vi "Highlighted Table  rows.vi"(8 "error in":errorcluster, 10 "Number of highlighted rows":i32, 11 "Tolerance Limits Listbox":refnum<vi>) -> (0 "error out":errorcluster)   [LabVIEW 2015, in "ZenGage v3.0 UI.lvclass"]
uses:
  ZenGage v3.0 UI.lvclass
  <vilib>/Utility/miscctls.llb/LVRowAndColumnTypeDef.ctl
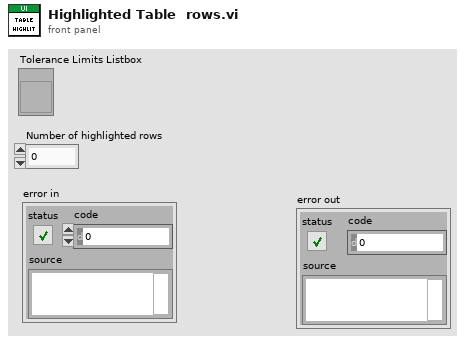
[diagram p1: front panel]
types:
  T1 = typedef "LVRowAndColumnTypeDef.ctl" = cluster{"Row":i32, "Column":i32}
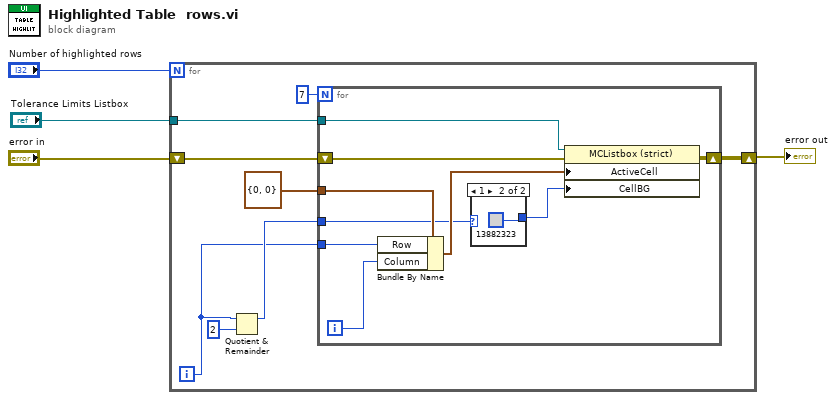
[diagram p0: block diagram]
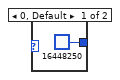
[diagram p2: hidden frame]
diagram:
  n1 = for {
    N: "Number of highlighted rows" -> [_]
    shift-right: [w10] -> w3
    shift-left: "error in" -> [w9]
    tunnel: "Tolerance Limits Listbox" -> [w6]
    i -> [w7]
    n2 = Quotient & Remainder(x=w7, y=2) -> (x-y*floor(x/y)=w8:i32)  [unwired: 1 out]
    n3 = for {
      N: 7 -> [_]
      tunnel: T1 {"Row"=0, "Column"=0} ("Active Cell:Active Cell") -> [w21]
      tunnel: w8 -> [w17]
      tunnel: w7 -> [w15]
      tunnel: w6 -> [w14]
      shift-right: [w19] -> w10
      shift-left: w9 -> [w18]
      i -> [w13]
      n4 = Bundle By Name(cluster=w21, "Row"=w15, "Column"=w13) -> (w20:T1)
      n5 = case shown="1" w17 {
        tunnel: [u32 16448250 u32 13882323] -> w16
        frame 0, Default {
        }
        frame 1 {
        }
      }
      n6 = property on="Property Node" class="MCListbox (strict)"(reference=w14, error in=w18, "ActiveCell"=w20, "CellBG"=w16) -> (error out=w19:errorcluster)  [unwired: 1 out]
    }
  }
  "error out" <- w3
